vi "TEST_MoveImage.vi"() -> ()   [LabVIEW 2021, in "Picture2D.lvlib"]
uses:
  Picture2D/Picture2D.lvlib
  Picture/Image.lvclass
  Point/Point.lvclass
panel:
  in  "stop":bool
  in  "Point:ToMove":cluster{"x":i16, "y":i16}={"x"=-10, "y"=-10} {"x" scale=-100.0..100.0; "y" scale=-100.0..100.0}
  in  "Absolute":bool
  out "2D Picture":picture
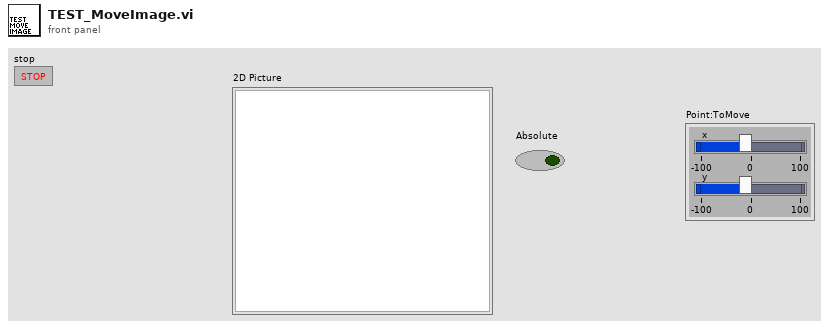
[diagram p1: front panel]
types:
  T1 = typedef "imagedata.ctl" = cluster{"image type":i32, "image depth":i32, "image":u8[], "mask":u8[], "colors":u32[], "Rectangle":cluster{"left":i16, "top":i16, "right":i16, "bottom":i16}}
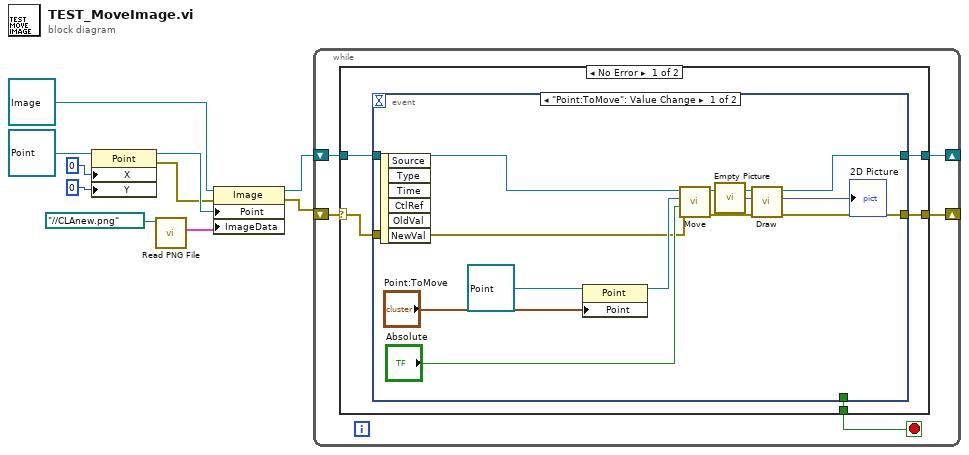
[diagram p0: block diagram]
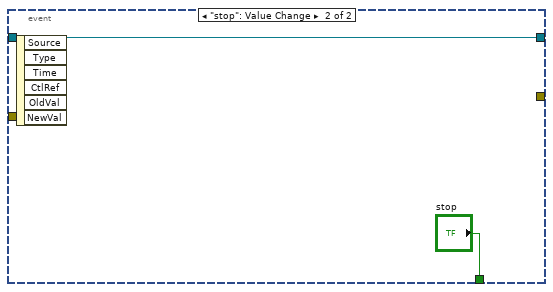
[diagram p2: hidden frame]
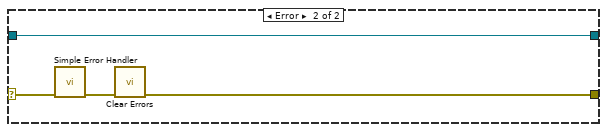
[diagram p3: hidden frame]
diagram:
  n1 = property class="Point"(reference=refnum<class "Point.lvclass"> refnum ("Point"), "X"=i16 0 ("Point:x"), "Y"=i16 0 ("Point:y")) -> (reference out=w6:refnum<class "Point.lvclass">, error out=w1:errorcluster)  [unwired: 1 in]
  n2 = call <vilib>:"Read PNG File.vi"("path to PNG file"=path "../../CLAnew.png") -> ("image data"=w8:T1)  [unwired: 8 in, 2 out]
  n3 = property class="Image"(reference=refnum<class "Image.lvclass"> refnum ("Image"), error in=w1, "Point"=w6, "ImageData"=w8) -> (reference out=w3:refnum<class "Image.lvclass">, error out=w2:errorcluster)
  n4 = while {
    shift-right: [w14] -> _
    shift-left: w3 -> [w13]
    shift-right: [w12] -> _
    shift-left: w2 -> [w11]
    stop <- w15 stop-if-true
    n5 = case shown="No Error" w11 {
      selector: w11 -> [w16 w38]
      tunnel: [w20 _] -> w15
      tunnel: [w19 w35] -> w14
      tunnel: w13 -> [w18 w35]
      tunnel: [w17 w36] -> w12
      frame No Error {
        n6 = event shown="[0] \"Point:ToMove\": Value Change" {
          selector: _ -> [_ _]
          dyn-events: _ -> [_ _]
          timeout: _ -> [_ _]
          tunnel: [_ "stop"] -> w20
          tunnel: [w25 w33] -> w19
          tunnel: w18 -> [w24 w33]
          tunnel: [w22 _] -> w17
          tunnel: w16 -> [w21 _]
          event "Point:ToMove": Value Change {
            n7 = event-data() -> ()  [unwired: 1 in, 6 out]
            n8 = property class="Point"(reference=refnum<class "Point.lvclass"> refnum ("Point"), "Point"="Point:ToMove") -> (reference out=w26:refnum<class "Point.lvclass">)  [unwired: 1 in, 1 out]
            n9 = call-dynamic "Move.vi"("error in (no error)"=w21, "Absolute (T)"="Absolute", "Point"=w26, "Image in"=w24) -> ("error out"=w23:errorcluster, "Image out"=w30:refnum<class "Image.lvclass">)  [unwired: 6 in]
            n10 = call "Empty Picture"() -> ("empty picture"=w32:picture)
            n11 = call-dynamic "Draw.vi"("error in (no error)"=w23, "2D Picture in"=w32, "Picture in"=w30) -> ("error out"=w22:errorcluster, "2D Picture out"=→"2D Picture":picture, "Picture out"=w25:refnum<class "Image.lvclass">)  [unwired: 6 in]
          }
          event "stop": Value Change {
            n12 = event-data() -> ()  [unwired: 1 in, 6 out]
          }
        }
      }
      frame Error {
        n13 = call <vilib>:"Simple Error Handler.vi"("error in (no error)"=w38) -> ("error out"=w37:errorcluster)  [unwired: 4 in, 4 out]
        n14 = call <vilib>:"Clear Errors.vi"("error in (no error)"=w37) -> ("error out"=w36:errorcluster)  [unwired: 5 in, 1 out]
      }
    }
  }
